vi "gl_UI Parameters.vi"() -> ()   [LabVIEW 2020]
panel:
  in  "global_UI Parameters":T1={"Z Start"=0.0, "Z Stop"=0.0, "Z Step"=1.0, "Pockels\n@Z Start"=0, "Pockels\n@Z Stop"=0, "# Planes"=0, "Dwell\nTime"=1.0, "Zoom"=1, "# Averaged Frames"=1, "PMT 2"=0, "PMT 1"=0, "Laser"=0, "AOL Z"=0.0, "Objective"="Olympus  20X", "Frame Size"=200, "AOL Mode"=1, "Field of View"=0} {"Field of View" items=["175", "235", "350"]; "AOL Mode" items=["Raster Scanning", "Structural Imaging", "Alignment Mode"]; "Frame Size" items=["20X20"=0, "100X100"=100, "128X128"=128, "200X200"=200, "256X256"=256, "512X512"=512]; "AOL Z" min=-115.4 max=130.2 step=0.01 scale=-115.4..130.2 scale format="%#_2f"; "Laser" max=100 step=1 scale=0.0..100.0; "PMT 1" min=0 max=1000 step=1 scale=0.0..1000.0; "PMT 2" min=0 max=1000 step=1 scale=0.0..1000.0; "# Averaged Frames" max=64 step=1; "Zoom" min=0 max=100 step=1 scale=0.0..100.0; "Dwell\nTime" min=0.08 max=12 step=0.08 scale=0.08..12.0}
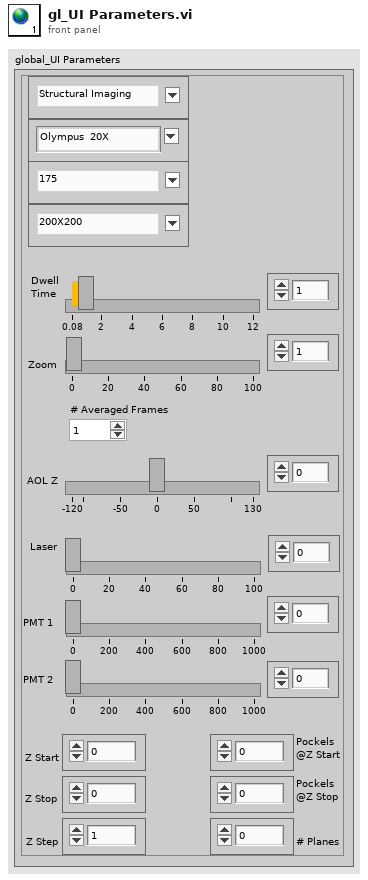
[diagram p1: front panel]
types:
  T1 = cluster{"Z Start":dbl, "Z Stop":dbl, "Z Step":dbl, "Pockels\n@Z Start":u8, "Pockels\n@Z Stop":u8, "# Planes":u16, "Dwell\nTime":sgl, "Zoom":i8, "# Averaged Frames":u16, "PMT 2":i16, "PMT 1":i16, "Laser":u8, "AOL Z":sgl, "Objective":string, "Frame Size":u16, "AOL Mode":u16, "Field of View":u16}
diagram:
